vi "Get Timestamp Text.vi"(1 "Module Init Timestamp":timestamp, 2 "Error Timestamp":timestamp) -> (0 "Timestamp String":string)   [LabVIEW 2016, in "Error Manager.lvlib"]
doc: "This VI generates a \"Timestamp String\", which can be displayed to the user and/or logged to the error log file."
uses:
  Error Manager.lvlib
panel:
  # "Development\nControls or indicators that are useful for development or testing, but which are not outputs of the VI."
  # "Input\nInputs to the VI"
  # "Output\nOutputs of the VI"
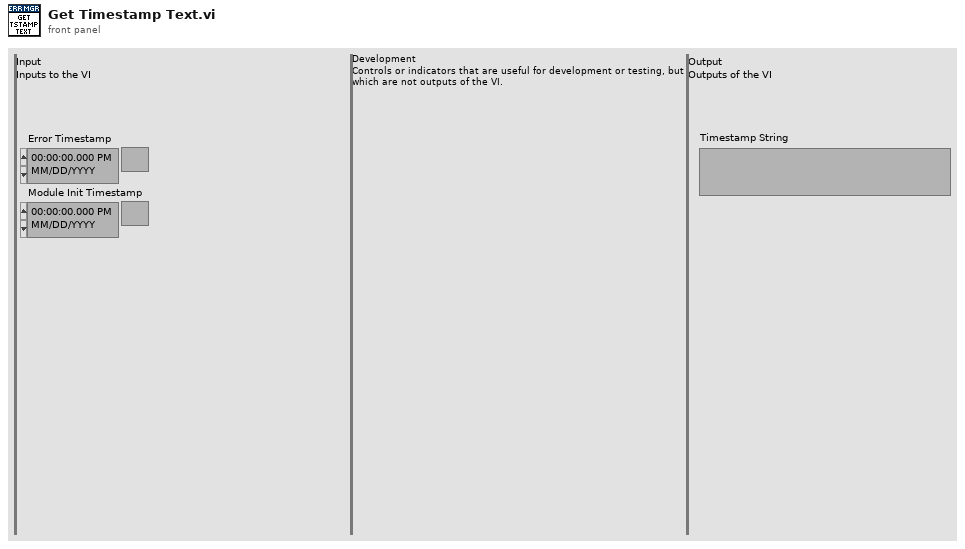
[diagram p1: front panel]
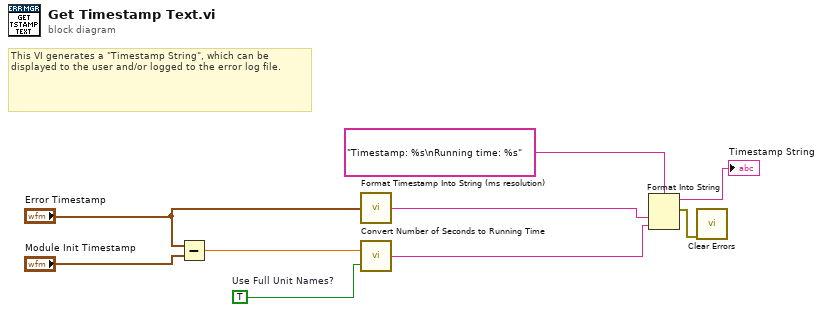
[diagram p0: block diagram]
diagram:
  w8 = TRUE  # Use Full Unit Names?
  # "This VI generates a \"Timestamp String\", which can be displayed to the user and/or logged to the error log file."
  n1 = Subtract(x="Error Timestamp", y="Module Init Timestamp") -> (x-y=w7:dbl)
  n2 = call "Format Timestamp Into String (ms resolution).vi"("Timestamp"="Error Timestamp") -> ("Timestamp String (ms resolution)"=w5:string)
  n3 = call "Convert Number of Seconds to Running Time.vi"("Use Full Unit Names? (F)"=w8, "Number of seconds elapsed"=w7) -> ("Running Time String"=w3:string)
  n4 = Format Into String(format string="Timestamp: %s\nRunning time: %s", w5, w3) -> (resulting string=→"Timestamp String":string, error out=w1:errorcluster)  [unwired: 2 in]
  n5 = call <vilib>:"Clear Errors.vi"("error in (no error)"=w1) -> ()  [unwired: 5 in, 2 out]
